vi "FTW-Project-CreateValidProjectRef.vi"(0 "Project Ref (blank for Active Project)":refnum<vi>, 11 "error in":errorcluster) -> (4 "Project Ref":refnum<vi>, 6 "Name":string, 15 "error out":errorcluster)   [LabVIEW 2012]
panel:
  # "Inputs"
  # "Outputs"
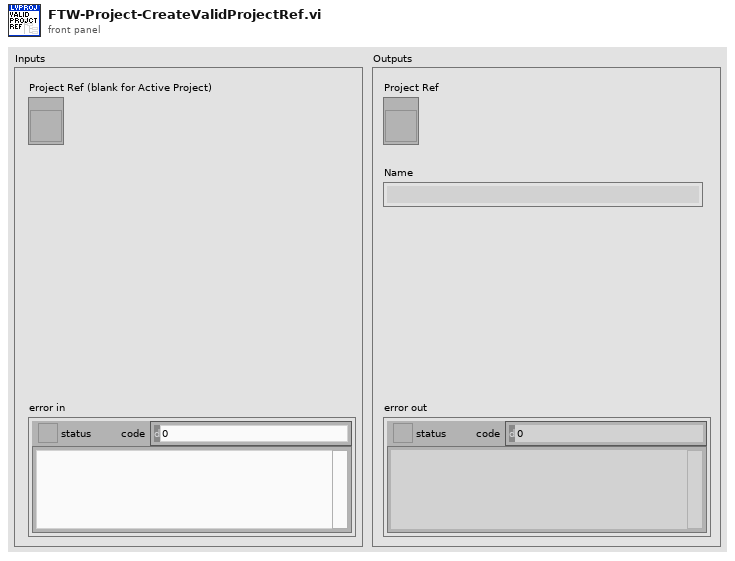
[diagram p1: front panel]
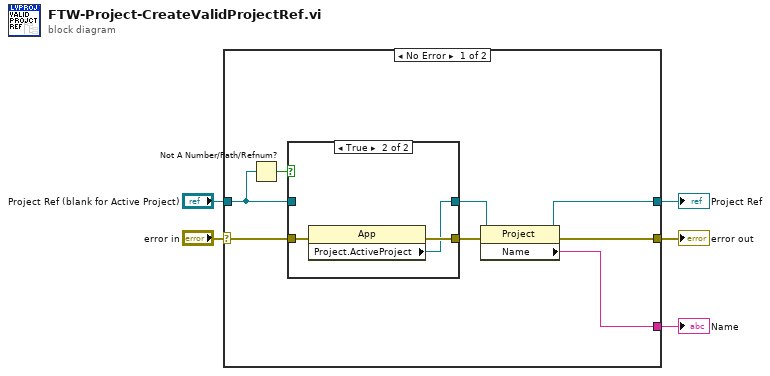
[diagram p0: block diagram]
diagram:
  n1 = case shown="No Error" "error in" {
    selector: "error in" -> [w13 w20]
    tunnel: [w7 w20] -> w5
    tunnel: "Project Ref (blank for Active Project)" -> [w9 w19]
    tunnel: [w8 w19] -> w2
    tunnel: [w6 _] -> w1
    frame No Error {
      n2 = Not A Number/Path/Refnum?(number/path/refnum=w9) -> (NaN/Path/Refnum?=w10:bool)
      n3 = case shown="True" w10 {
        tunnel: w13 -> [w14 w18]
        tunnel: [w14 w17] -> w12
        tunnel: [w15 w16] -> w11
        tunnel: w9 -> [w15 _]
        frame False {
        }
        frame True {
          n4 = property class="App"(error in=w18) -> (error out=w17:errorcluster, "Project.ActiveProject"=w16:refnum<vi>)  [unwired: 1 in, 1 out]
        }
      }
      n5 = property class="Project"(reference=w11, error in=w12) -> (reference out=w8:refnum<vi>, error out=w7:errorcluster, "Name"=w6:string)
    }
    frame Error {
    }
  }
  "error out" <- w5
  "Project Ref" <- w2
  "Name" <- w1
